vi "VI Tree.vi"   [LabVIEW 2013, in "Yokogawa WT200 Series.lvlib"]
doc: "This is the instrument driver for the WT200 Series. The VI Tree displays all the user-callable VIs of the instrument driver in an organized table.\n\nThis Instrument Driver's Revision number is 1.10 and is compatible with Instrument Firmware Revision F3.11(WT200), F1.06(WT210/WT230)\n\nYOKOGAWA WT200/WT210/WT230 Digital Power Meter\nCreated By: Yokogawa Electric Corporation\nRelease Date: 09/2002\nOriginally Developed in LabVIEW Version: 5.0.1\n\nNOTE : This insturument driver use the communication commands conforming to the IEEE 488.2 Standard."
uses:
  <instrlib>/Yokogawa WT200 Series/Yokogawa WT200 Series.lvlib
panel:
  # "© 2005 National Instruments.  ALL RIGHTS RESERVED."
  # "SEE DIAGRAM\nFOR VI TREE."
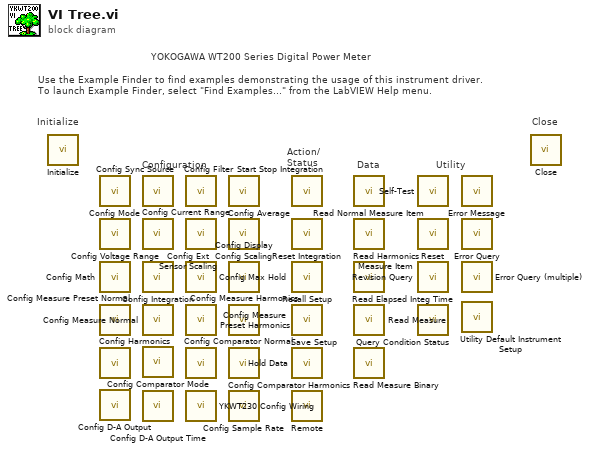
[diagram p0: block diagram]
diagram:
  # "YOKOGAWA WT200 Series Digital Power Meter"
  # "Use the Example Finder to find examples demonstrating the usage of this instrument driver.\nTo launch Example Finder, select \"Find Examples...\" from the LabVIEW Help menu."
  # "Configuration"
  # "Utility"
  # "Data"
  # "Action/\nStatus"
  # "Close"
  # "Initialize"
  n1 = call <instrlib>:"Initialize.vi"() -> ()  [unwired: 14 in, 2 out]
  n2 = call <instrlib>:"Config Mode.vi"() -> ()  [unwired: 14 in, 2 out]
  n3 = call <instrlib>:"Config Voltage Range.vi"() -> ()  [unwired: 14 in, 2 out]
  n4 = call <instrlib>:"Config Math.vi"() -> ()  [unwired: 14 in, 2 out]
  n5 = call <instrlib>:"Config Measure Preset Normal.vi"() -> ()  [unwired: 14 in, 2 out]
  n6 = call <instrlib>:"Config Harmonics.vi"() -> ()  [unwired: 14 in, 2 out]
  n7 = call <instrlib>:"Config D-A Output.vi"() -> ()  [unwired: 14 in, 2 out]
  n8 = call <instrlib>:"Config Sync Source.vi"() -> ()  [unwired: 14 in, 2 out]
  n9 = call <instrlib>:"Config Current Range.vi"() -> ()  [unwired: 14 in, 2 out]
  n10 = call <instrlib>:"Config Integration.vi"() -> ()  [unwired: 14 in, 2 out]
  n11 = call <instrlib>:"Config Measure Normal.vi"() -> ()  [unwired: 14 in, 2 out]
  n12 = call <instrlib>:"Config Comparator Mode.vi"() -> ()  [unwired: 14 in, 2 out]
  n13 = call <instrlib>:"Config D-A Output Time.vi"() -> ()  [unwired: 14 in, 2 out]
  n14 = call <instrlib>:"Config Filter.vi"() -> ()  [unwired: 14 in, 2 out]
  n15 = call <instrlib>:"Config Ext Sensor Scaling.vi"() -> ()  [unwired: 14 in, 2 out]
  n16 = call <instrlib>:"Config Max Hold.vi"() -> ()  [unwired: 14 in, 2 out]
  n17 = call <instrlib>:"Config Measure Preset Harmonics.vi"() -> ()  [unwired: 14 in, 2 out]
  n18 = call <instrlib>:"Config Comparator Normal.vi"() -> ()  [unwired: 14 in, 2 out]
  n19 = call <instrlib>:"YKWT230 Config Wiring.vi"() -> ()  [unwired: 14 in, 2 out]
  n20 = call <instrlib>:"Config Average.vi"() -> ()  [unwired: 14 in, 2 out]
  n21 = call <instrlib>:"Config Scaling.vi"() -> ()  [unwired: 14 in, 2 out]
  n22 = call <instrlib>:"Config Display.vi"() -> ()  [unwired: 14 in, 2 out]
  n23 = call <instrlib>:"Config Measure Harmonics.vi"() -> ()  [unwired: 14 in, 2 out]
  n24 = call <instrlib>:"Config Comparator Harmonics.vi"() -> ()  [unwired: 14 in, 2 out]
  n25 = call <instrlib>:"Config Sample Rate.vi"() -> ()  [unwired: 14 in, 2 out]
  n26 = call <instrlib>:"Start Stop Integration.vi"() -> ()  [unwired: 14 in, 2 out]
  n27 = call <instrlib>:"Reset Integration.vi"() -> ()  [unwired: 14 in, 2 out]
  n28 = call <instrlib>:"Recall Setup.vi"() -> ()  [unwired: 14 in, 2 out]
  n29 = call <instrlib>:"Save Setup.vi"() -> ()  [unwired: 14 in, 2 out]
  n30 = call <instrlib>:"Hold Data.vi"() -> ()  [unwired: 14 in, 2 out]
  n31 = call <instrlib>:"Remote.vi"() -> ()  [unwired: 14 in, 2 out]
  n32 = call <instrlib>:"Read Normal Measure Item.vi"() -> ()  [unwired: 12 in, 4 out]
  n33 = call <instrlib>:"Read Harmonics Measure Item.vi"() -> ()  [unwired: 13 in, 3 out]
  n34 = call <instrlib>:"Read Elapsed Integ Time.vi"() -> ()  [unwired: 11 in, 5 out]
  n35 = call <instrlib>:"Read Measure.vi"() -> ()  [unwired: 12 in, 4 out]
  n36 = call <instrlib>:"Read Measure Binary.vi"() -> ()  [unwired: 8 in, 8 out]
  n37 = call <instrlib>:"Self-Test.vi"() -> ()  [unwired: 12 in, 4 out]
  n38 = call <instrlib>:"Reset.vi"() -> ()  [unwired: 14 in, 2 out]
  n39 = call <instrlib>:"Revision Query.vi"() -> ()  [unwired: 12 in, 4 out]
  n40 = call <instrlib>:"Query Condition Status.vi"() -> ()  [unwired: 13 in, 3 out]
  n41 = call <instrlib>:"Error Message.vi"() -> ()  [unwired: 11 in, 5 out]
  n42 = call <instrlib>:"Error Query.vi"() -> ()  [unwired: 12 in, 4 out]
  n43 = call <instrlib>:"Error Query (multiple).vi"() -> ()  [unwired: 12 in, 4 out]
  n44 = call <instrlib>:"Utility Default Instrument Setup.vi"() -> ()  [unwired: 14 in, 2 out]
  n45 = call <instrlib>:"Close.vi"() -> ()  [unwired: 15 in, 1 out]
